vi "max research V2.vi"() -> ()   [LabVIEW 2023]
panel:
  in  "?":bool
  out "?":bool
  out "min research":dbl
  out "Waveform Chart":dbl(graph)
  out "current iteration":i32
  out "max research":dbl
  in  "number of iteration":i32
  out "latest value":dbl
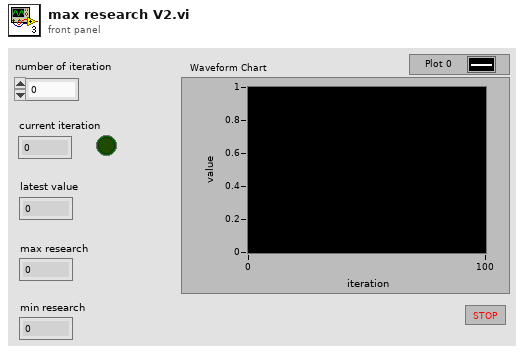
[diagram p1: front panel]
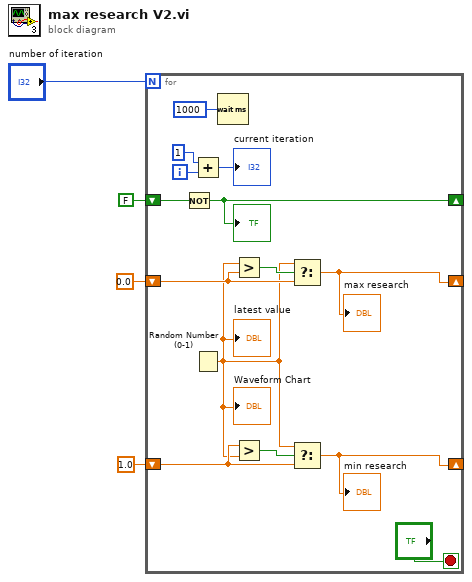
[diagram p0: block diagram]
diagram:
  n1 = for {
    N: "number of iteration" -> [_]
    shift-right: [w18] -> _
    shift-left: 0.0 ("number: 0 to 1") -> [w9]
    shift-right: [w15] -> _
    shift-left: FALSE -> [w16]
    shift-right: [w6] -> _
    shift-left: 1.0 ("number: 0 to 1") -> [w7]
    i -> [w17]
    stop <- "?" stop-if-true
    n2 = Not(x=w16) -> (.not. x?=w15:bool)
    "?" <- w15
    n3 = Add(x=1, y=w17) -> (x+y=→"current iteration":i32)
    n4 = Random Number (0-1)() -> (number: 0 to 1=w5:dbl)
    "latest value" <- w5
    "Waveform Chart" <- w5
    n5 = Wait (ms)(milliseconds to wait=u32 1000) -> ()  [unwired: 1 out]
    n6 = Greater?(x=w5, y=w9) -> (0:w10:bool)
    n7 = Greater?(x=w7, y=w5) -> (0:w8:bool)
    n8 = Select(t=w5, s=w10, f=w9) -> (s? t:f=w18:dbl)
    "max research" <- w18
    n9 = Select(t=w5, s=w8, f=w7) -> (s? t:f=w6:dbl)
    "min research" <- w6
  }
